vi "校准Main.vi"() -> ()   [LabVIEW 2022 SP3, in "斯坦道多参数.lvlib"]
uses:
  <vilib>/ErrorRing/Error Ring.xnode
  <vilib>/ptbypt/NI_PtbyPt.lvlib
panel:
  in  "校准参数":u16(ring) caption="校准参数：" items=["pH"=0, "DO"=1, "浊度"=2, "电导率"=3, "余氯"=13]
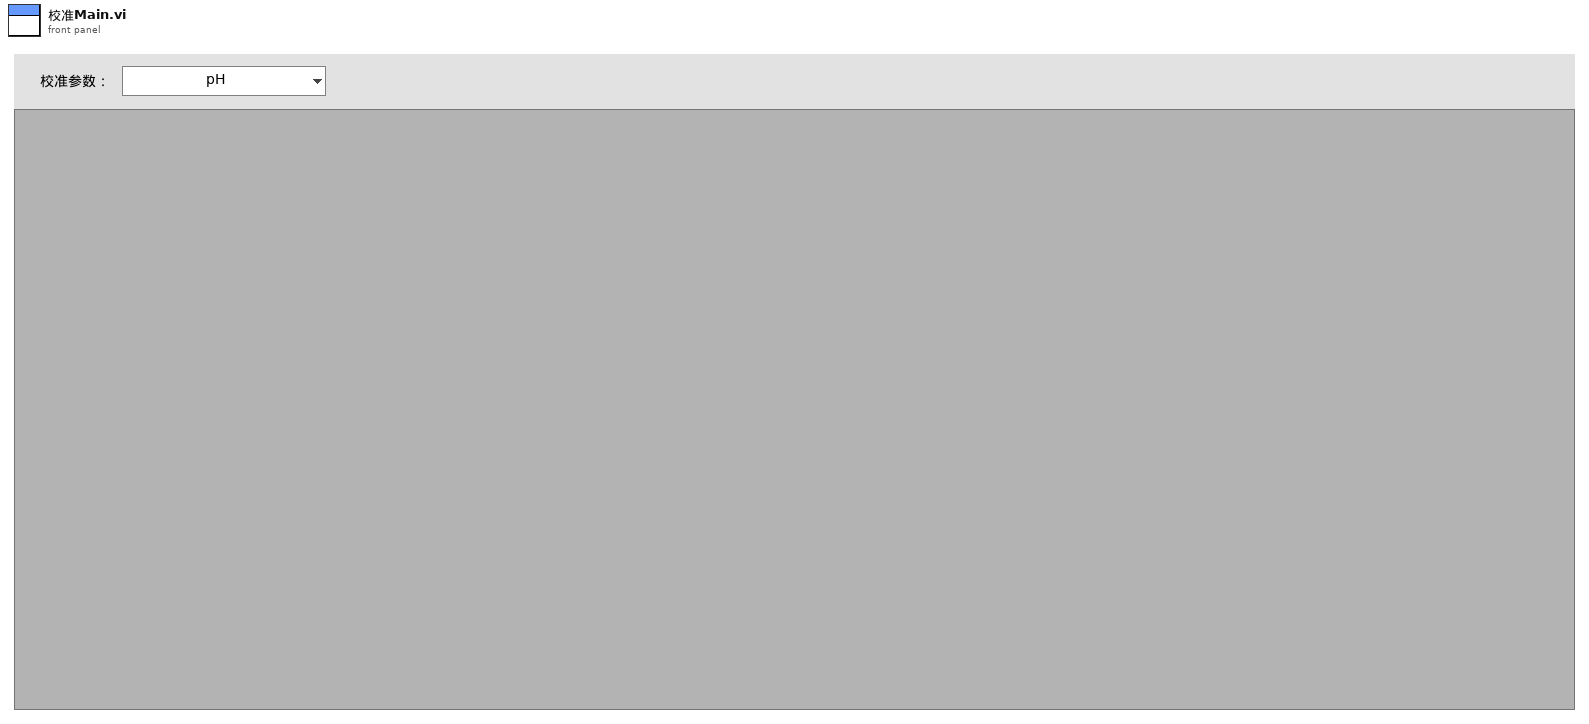
[diagram p1: front panel]
types:
  T1 = typedef "LVStringsAndValuesArrayTypeDef_U16.ctl" = cluster{"String":string, "Value":u16}[]
  T2 = enum32{"Bad", "Idle", "Run top level", "Running"}
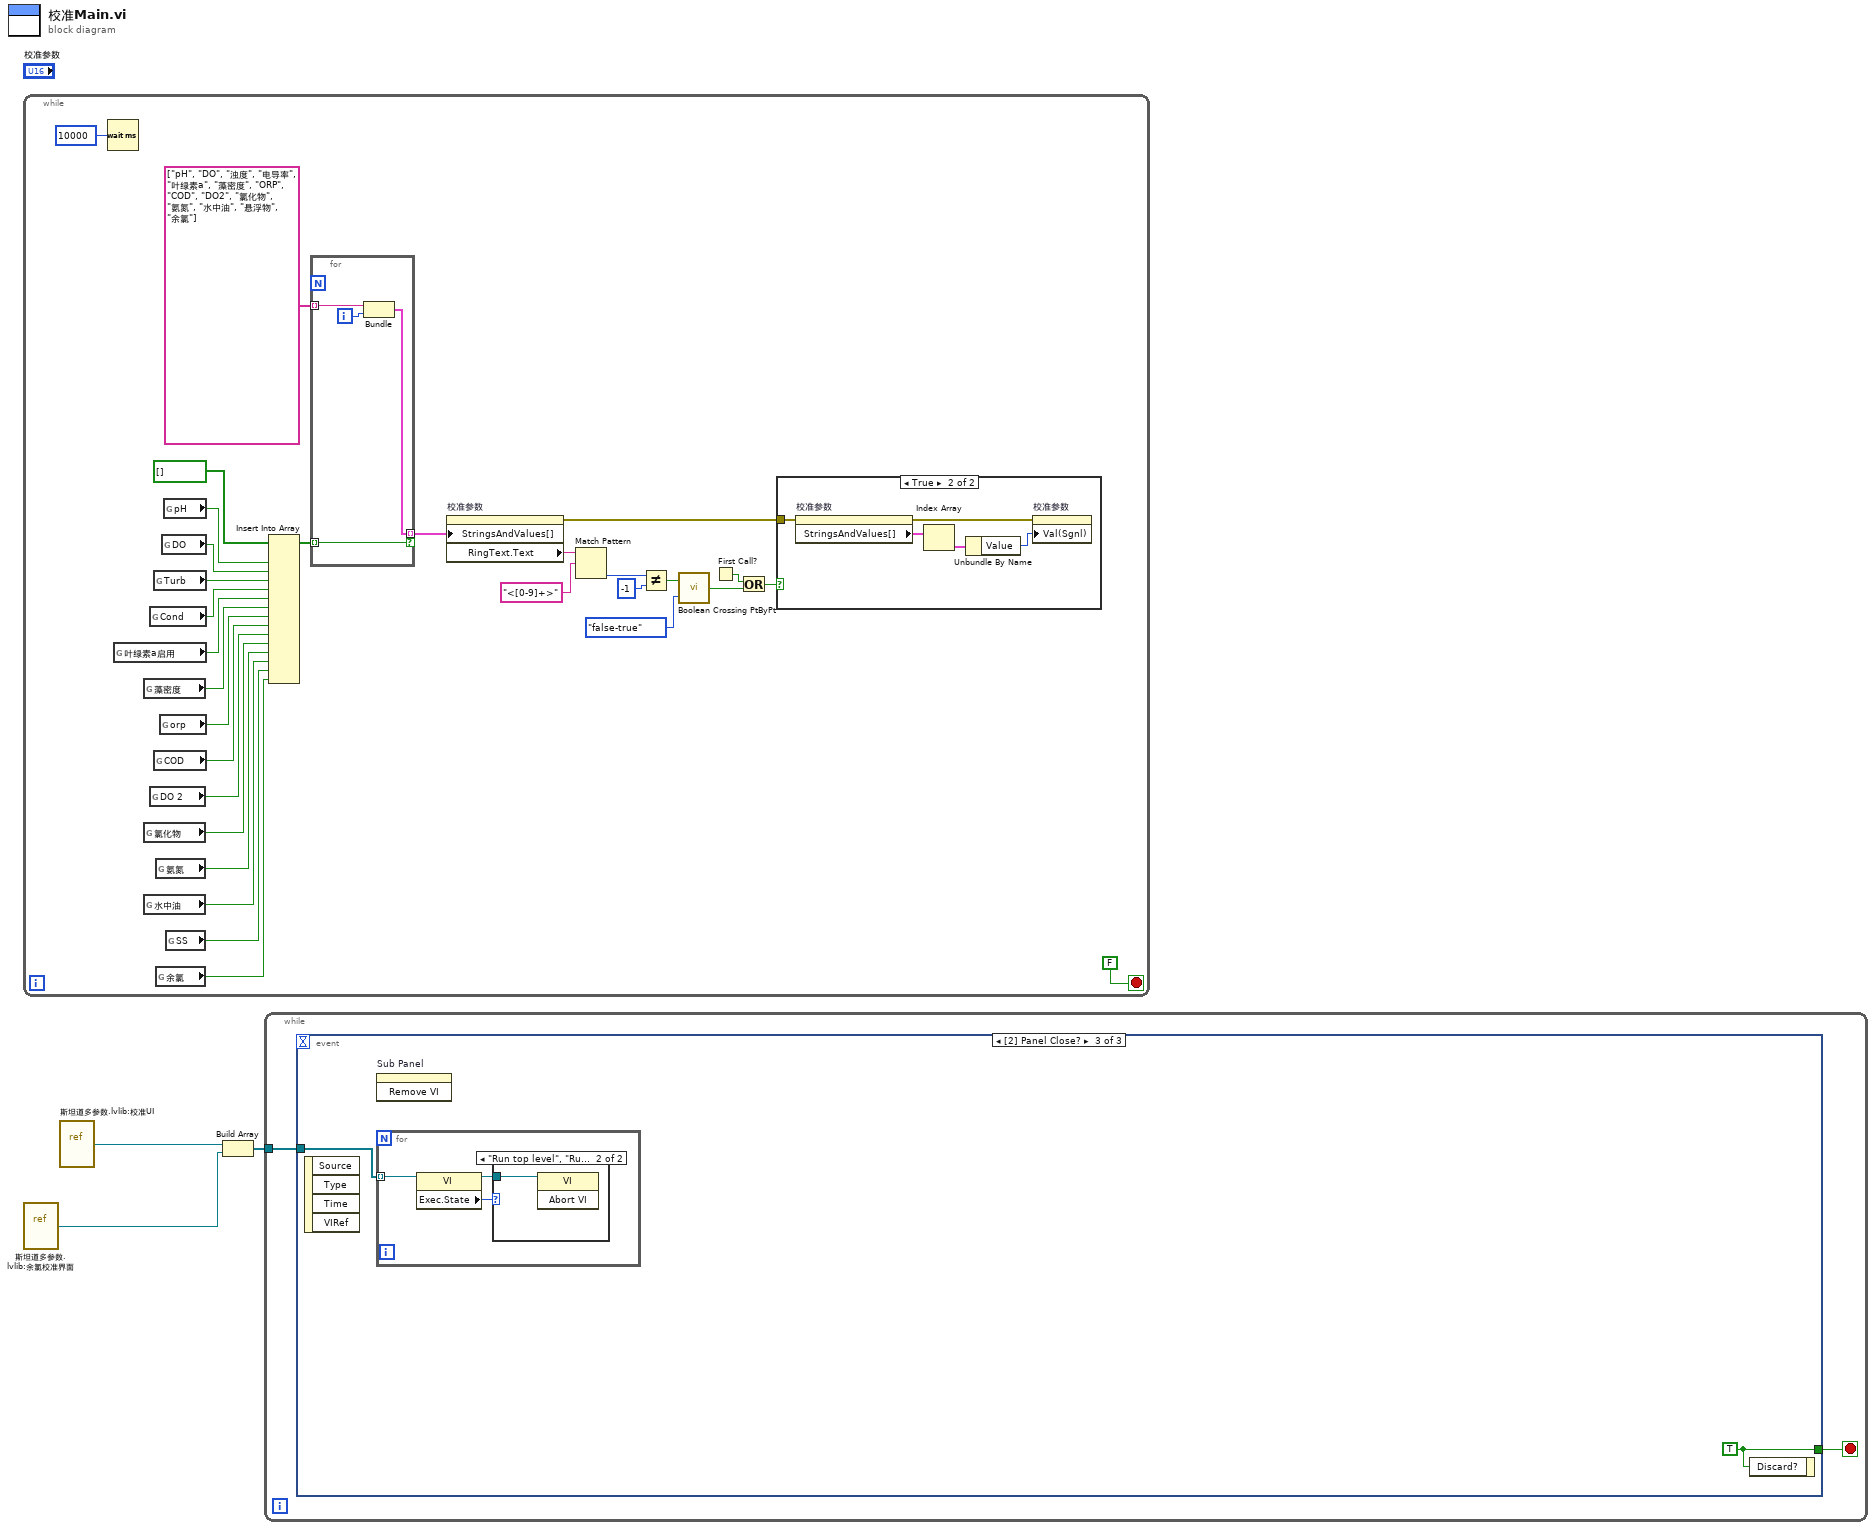
[diagram p0: block diagram]
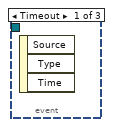
[diagram p2: hidden frame]
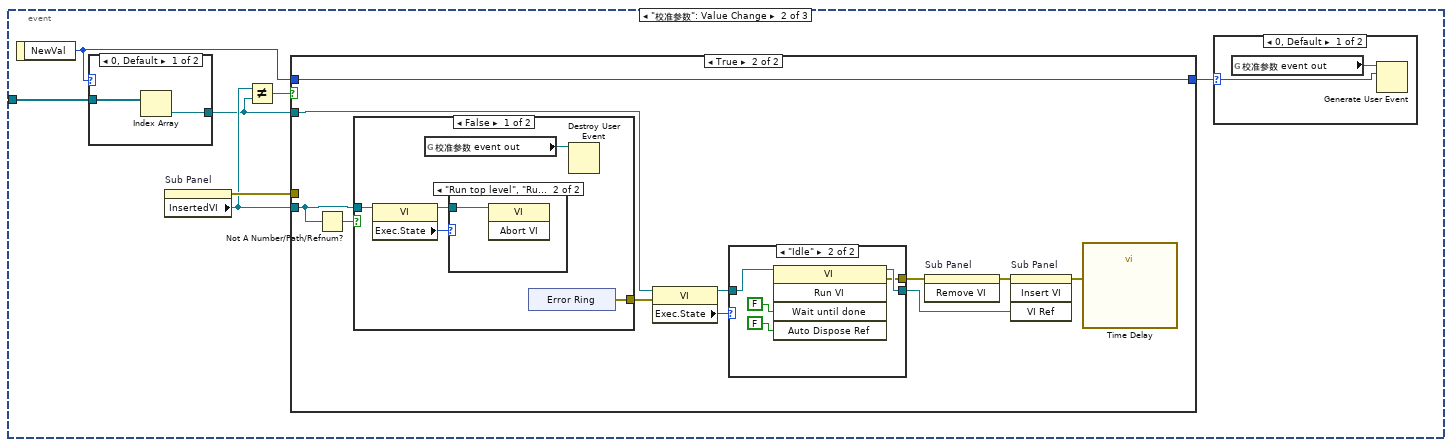
[diagram p3: hidden frame]
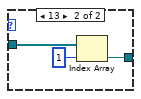
[diagram p9: hidden frame]
diagram:
  n1 = while {
    stop <- FALSE stop-if-true
    n2 = Wait (ms)(milliseconds to wait=u32 10000 ("等待时间（毫秒）")) -> ()  [unwired: 1 out]
    n3 = global read "断电保存变量.vi" "叶绿素a启用"() -> (w13:bool)
    n4 = global read "断电保存变量.vi" "藻密度"() -> (w12:bool)
    n5 = global read "断电保存变量.vi" "氯化物"() -> (w8:bool)
    n6 = global read "断电保存变量.vi" "水中油"() -> (w6:bool)
    n7 = global read "断电保存变量.vi" "Cond"() -> (w14:bool)
    n8 = global read "断电保存变量.vi" "DO 2"() -> (w9:bool)
    n9 = global read "断电保存变量.vi" "Turb"() -> (w30:bool)
    n10 = global read "断电保存变量.vi" "COD"() -> (w10:bool)
    n11 = global read "断电保存变量.vi" "氨氮"() -> (w7:bool)
    n12 = global read "断电保存变量.vi" "余氯"() -> (w4:bool)
    n13 = global read "断电保存变量.vi" "orp"() -> (w11:bool)
    n14 = global read "断电保存变量.vi" "DO"() -> (w31:bool)
    n15 = global read "断电保存变量.vi" "pH"() -> (w33:bool)
    n16 = global read "断电保存变量.vi" "SS"() -> (w5:bool)
    n17 = Insert Into Array(array=bool[] [] ("数组"), new element #1=w33, new element #2=w31, new element #3=w30, new element #4=w14, new element #5=w13, new element #6=w12, new element #7=w11, new element #8=w10, new element #9=w9, new element #10=w8, new element #11=w7, new element #12=w6, new element #13=w5, new element #14=w4) -> (w27:bool[])  [unwired: 1 in]
    n18 = for {
      tunnel: w27 -> [w39] mode=indexing
      tunnel: string[] ["pH", "DO", "浊度", "电导率", "叶绿素a", "藻密度", "ORP", "COD", "DO2", "氯化物", "氨氮", "水中油", "悬浮物", "余氯"] ("字符串[]") -> [w41] mode=indexing
      tunnel: [w40] -> w24 mode=indexing if=w39
      i -> [w42]
      n19 = Bundle(w41, w42) -> (w40:cluster{string, i32})  [unwired: 1 in]
    }
    n20 = property on="校准参数" class="Ring (strict)"("StringsAndValues[]"=w24) -> (error out=w25:errorcluster, "RingText.Text"=w23:string)  [unwired: 2 in, 1 out]
    n21 = Match Pattern(string=w23, regular expression="<[0-9]+>" ("正则表达式")) -> (offset past match=w21:i32)  [unwired: 1 in, 3 out]
    n22 = Not Equal?(x=w21, y=-1) -> (x != y?=w19:bool)
    n23 = call <vilib>:"Boolean Crossing PtByPt.vi"("direction"=enum16{"either", "false-true", "true-false"}."false-true", "input"=w19) -> ("crossing"=w16:bool)  [unwired: 1 in]
    n24 = First Call?() -> (First Call?: T/F=w17:bool)
    n25 = Or(x=w17, y=w16) -> (x .or. y?=w18:bool)
    n26 = case shown="True" w18 {
      tunnel: w25 -> [_ w38]
      frame False {
      }
      frame True {
        n27 = property on="校准参数" class="Ring (strict)"(error in=w38) -> (error out=w37:errorcluster, "StringsAndValues[]"=w36:T1)  [unwired: 1 in, 1 out]
        n28 = Index Array(array=w36) -> (element=w35:cluster{"String":string, "Value":u16})  [unwired: 1 in]
        n29 = Unbundle By Name(w35) -> ("Value"=w34:u16)
        n30 = property on="校准参数" class="Ring (strict)"(error in=w37, "Val(Sgnl)"=w34) -> ()  [unwired: 1 in, 2 out]
      }
    }
  }
  n31 = vi-ref "斯坦道多参数.lvlib:余氯校准界面.vi"() -> (w3:refnum<vi>)
  n32 = vi-ref "斯坦道多参数.lvlib:校准UI.vi"() -> (w1:refnum<vi>)
  n33 = Build Array(w1, w3) -> (w2:refnum<vi>[])
  n34 = while {
    tunnel: w2 -> [w44]
    stop <- w43 stop-if-true
    n35 = event shown="[2] Panel Close?" {
      selector: _ -> [_ _ _]
      dyn-events: _ -> [_ _ _]
      timeout: _ -> [_ _ _]
      tunnel: w44 -> [_ w51 w84]
      tunnel: [_ _ w85] -> w43
      event Timeout {
        n36 = event-data() -> ()  [unwired: 1 in, 3 out]
      }
      event "校准参数": Value Change {
        n37 = event-data() -> ("NewVal"=w45:u16)  [unwired: 1 in]
        n38 = case shown="0, Default" w45 {
          tunnel: w51 -> [w80 w83]
          tunnel: [w79 w81] -> w48
          frame 0, Default {
            n39 = Index Array(array=w80) -> (element=w79:refnum<vi>)  [unwired: 1 in]
          }
          frame 13 {
            n40 = Index Array(array=w83, index=1) -> (element=w81:refnum<vi>)
          }
        }
        n41 = property on="Sub Panel" class="SubPnl"() -> (error out=w50:errorcluster, "InsertedVI"=w49:refnum<vi>)  [unwired: 2 in, 1 out]
        n42 = Not Equal?(x=w49, y=w48) -> (x != y?=w47:bool)
        n43 = case shown="True" w47 {
          tunnel: w50 -> [_ _]
          tunnel: w49 -> [_ w58]
          tunnel: w48 -> [_ w61]
          tunnel: [w54 w59] -> w46
          tunnel: w45 -> [w54 w59]
          frame False {
          }
          frame True {
            n44 = Not A Number/Path/Refnum?(number/path/refnum=w58) -> (NaN/Path/Refnum?=w60:bool)
            n45 = case shown="False" w60 {
              tunnel: w58 -> [w66 _]
              tunnel: [w69 _] -> w56
              frame False {
                n46 = property class="VI"(reference=w66) -> (reference out=w67:refnum<vi>, "Exec.State"=w68:T2)  [unwired: 1 in, 1 out]
                n47 = global read "多参数全局变量.vi" "校准参数 event out"() -> (w70:refnum<user-event>)
                n48 = case shown="\"Run top level\", \"Running\"" w68 {
                  tunnel: w67 -> [_ w71]
                  frame "Bad", Default {
                  }
                  frame "Run top level", "Running" {
                    n49 = invoke class="VI" method="Abort VI"(reference=w71) -> ()  [unwired: 2 in, 3 out]
                  }
                }
                n50 = xnode "Error Ring"() -> ("error out"=w69:errorcluster)
                n51 = Destroy User Event(user event=w70) -> ()  [unwired: 1 in, 1 out]
              }
              frame True {
              }
            }
            n52 = property class="VI"(reference=w61, error in=w56) -> (reference out=w64:refnum<vi>, "Exec.State"=w65:T2)  [unwired: 1 out]
            n53 = case shown="\"Idle\"" w65 {
              tunnel: [w73 w76] -> w62
              tunnel: w64 -> [w73 w75]
              tunnel: [_ w74] -> w57
              frame "Bad", Default {
              }
              frame "Idle" {
                n54 = invoke class="VI" method="Run VI"(reference=w75, "Wait until done"=FALSE ("结束前等待"), "Auto Dispose Ref"=FALSE ("自动销毁引用")) -> (reference out=w76:refnum<vi>, error out=w74:errorcluster)  [unwired: 2 in, 3 out]
              }
            }
            n55 = invoke on="Sub Panel" class="SubPnl" method="Remove VI"(error in=w57) -> (error out=w63:errorcluster)  [unwired: 2 in, 2 out]
            n56 = invoke on="Sub Panel" class="SubPnl" method="Insert VI"(error in=w63, "VI Ref"=w62) -> (error out=w55:errorcluster)  [unwired: 2 in, 3 out]
            n57 = call "Time Delay"("error in (no error)"=w55) -> ()  [unwired: 10 in, 1 out]
          }
        }
        n58 = case shown="0, Default" w46 {
          selector: w46 -> [w52 _]
          frame 0, Default {
            n59 = global read "多参数全局变量.vi" "校准参数 event out"() -> (w53:refnum<user-event>)
            n60 = Generate User Event(user event=w53, event data cluster=w52) -> ()  [unwired: 2 in, 2 out]
          }
          frame 13 {
          }
        }
      }
      event Panel Close? {
        w85 = TRUE ("Discard?")
        n61 = event-data() -> ()  [unwired: 1 in, 4 out]
        n62 = invoke on="Sub Panel" class="SubPnl" method="Remove VI"() -> ()  [unwired: 3 in, 3 out]
        n63 = for {
          tunnel: w84 -> [w88] mode=indexing
          n64 = property class="VI"(reference=w88) -> (reference out=w86:refnum<vi>, "Exec.State"=w87:T2)  [unwired: 1 in, 1 out]
          n65 = case shown="\"Run top level\", \"Running\"" w87 {
            tunnel: w86 -> [_ w89]
            frame "Bad", Default {
            }
            frame "Run top level", "Running" {
              n66 = invoke class="VI" method="Abort VI"(reference=w89) -> ()  [unwired: 2 in, 3 out]
            }
          }
        }
        n67 = event-data("Discard?"=w85) -> ()  [unwired: 1 in, 1 out]
      }
    }
  }
